vi "dg535 set output.vi"(0 "VISA resource name":refnum<visa-resource-name>, 5 "error in":errorcluster, 6 "output":u16(ring) items=["T0", "A", "B", "AB", "C", "D", "CD"], 7 "amplitude":dbl=1.0 min=-3.0 max=4.0 format="%.2f", 8 "mode":i32(ring) items=["TTL", "NIM", "ECL", "VAR"], 9 "offset":dbl min=-3.0 max=4.0 format="%.2f", 10 "load":bool, 12 "inversion":bool) -> (14 "VISA resource out":refnum<visa-resource-name>, 19 "error out":errorcluster)   [LabVIEW 2011]
doc: "This subVI sets the mode , load , output polarity , amplitude and offset of an output BNC .\nOUTPUT selects the BNC whose parameters will be changed .\nMODE specifies the output mode to be one of TTL, NIM , ECL or VAR .\nLOAD configures the output to drive either a 50 Ohm load or a High Z load .\nINVERSION sets the polarity of logic pulses at the BNC outputs. \nAMPLITUDE and OFFSET set the size of the step and the offset of the output BNCs when in the VARiable mode ."
panel:
  # "50 Ohm\nHigh Z"
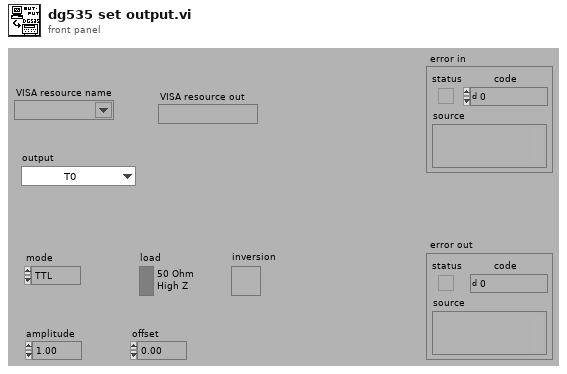
[diagram p1: front panel]
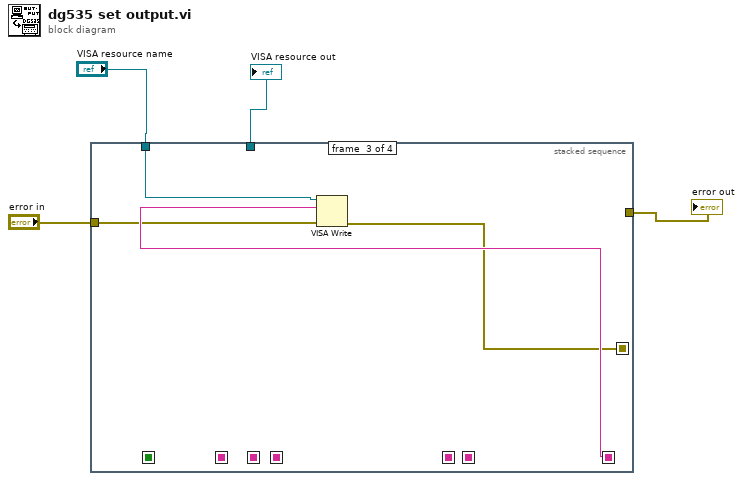
[diagram p0: block diagram]
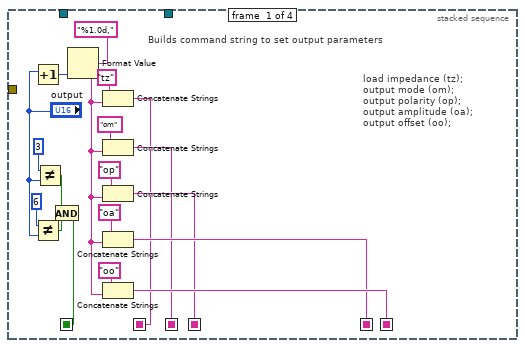
[diagram p2: hidden frame]
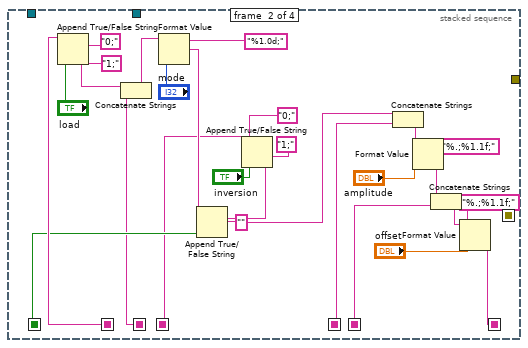
[diagram p3: hidden frame]
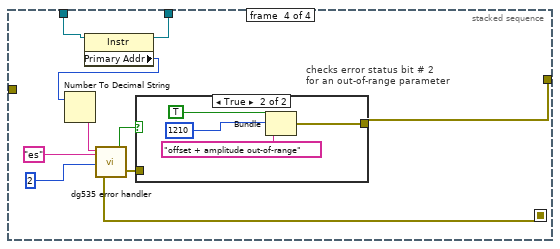
[diagram p4: hidden frame]
diagram:
  n1 = stacked-sequence {
    seq-local: [w16 _ _ _] -> [_ w29 _ _]
    seq-local: [w15 _ _ _] -> [_ w33 _ _]
    seq-local: [w14 _ _ _] -> [_ w30 _ _]
    seq-local: [w13 _ _ _] -> [_ w51 _ _]
    seq-local: [w17 _ _ _] -> [_ w39 _ _]
    seq-local: [w7 _ _ _] -> [_ w34 _ _]
    seq-local: [_ w27 _ _] -> [_ _ w55 _]
    seq-local: [_ _ w54 _] -> [_ _ _ w61]
    tunnel: "VISA resource name" -> [_ _ w52 w59]
    tunnel: "error in" -> [_ _ w53 _]
    tunnel: [_ _ _ w60] -> w3
    tunnel: [_ _ _ w58] -> w1
    frame #0 {
      # "load impedance (tz);\noutput mode (om);\noutput polarity (op);\noutput amplitude (oa);\noutput offset (oo);"
      # "Builds command string to set output parameters"
      n2 = Increment(x="output") -> (x+1=w12:u16)
      n3 = Not Equal?(x=6, y="output") -> (x != y?=w8:bool)
      n4 = Not Equal?(x=3, y="output") -> (x != y?=w9:bool)
      n5 = And(x=w9, y=w8) -> (x .and. y?=w7:bool)
      n6 = Format Value(format string="%1.0d,", value (0)=w12) -> (output string=w5:string)  [unwired: 1 in]
      n7 = Concatenate Strings("tz", w5) -> (w13:string)
      n8 = Concatenate Strings("om", w5) -> (w14:string)
      n9 = Concatenate Strings("op", w5) -> (w15:string)
      n10 = Concatenate Strings("oa", w5) -> (w16:string)
      n11 = Concatenate Strings("oo", w5) -> (w17:string)
    }
    frame #1 {
      n12 = Append True/False String(1:"load", 2:"1;", 3:"0;", 4:w51) -> (0:w46:string)
      n13 = Concatenate Strings(w46, w30) -> (w45:string)
      n14 = Format Value(string ("")=w45, format string="%1.0d;", value (0)="mode") -> (output string=w35:string)
      n15 = Append True/False String(1:"inversion", 2:"1;", 3:"0;", 4:w33) -> (0:w32:string)
      n16 = Append True/False String(1:w34, 2:"", 3:w32, 4:w35) -> (0:w28:string)
      n17 = Concatenate Strings(w28, w29) -> (w41:string)
      n18 = Format Value(string ("")=w41, format string="%.;%1.1f;", value (0)="amplitude") -> (output string=w38:string)
      n19 = Concatenate Strings(w38, w39) -> (w37:string)
      n20 = Format Value(string ("")=w37, format string="%.;%1.1f;", value (0)="offset") -> (output string=w27:string)
    }
    frame #2 {
      n21 = VISA Write(VISA resource name=w52, write buffer=w55, error in (no error)=w53) -> (error out=w54:errorcluster)  [unwired: 2 out]
    }
    frame #3 {
      # "checks error status bit # 2\nfor an out-of-range parameter"
      n22 = property class="Instr"(reference=w59) -> (reference out=w58:refnum<visa-resource-name>, "Primary Addr"=w57:u16)  [unwired: 1 in, 1 out]
      n23 = Number To Decimal String(number=w57) -> (decimal integer string=w56:string)  [unwired: 1 in]
      n24 = call "dg535 error handler.vi"("error in"=w61, "check bit #"=2, "command string"="es", "GPIB address"=w56) -> ("error out"=w62:errorcluster, "error found"=w63:bool)
      n25 = case shown="True" w63 {
        tunnel: [w66 w67] -> w60
        tunnel: w62 -> [w66 _]
        frame False {
        }
        frame True {
          n26 = Bundle(TRUE, 1210, "offset + amplitude out-of-range") -> (w67:errorcluster)  [unwired: 1 in]
        }
      }
    }
  }
  "error out" <- w3
  "VISA resource out" <- w1
